vi "fetch_and_translate_trigger.vi"(8 "error in (no error)":errorcluster, 11 "AnalyserDL090624Scaffold in":refnum<class "AnalyserDL090624Scaffold.lvclass">) -> (0 "error out":errorcluster, 1 "sender TLC type":T1=enum."ImagingMode", 2 "trigger":T2, 3 "AnalyserDL090624Scaffold out":refnum<class "AnalyserDL090624Scaffold.lvclass">)   [LabVIEW 2010, in "AnalyserDL090624Scaffold.lvclass"]
uses:
  AnalyserDL090624Scaffold.lvclass
  internal_trigger_enum.ctl
  common/enumerations/top-level_component_type_enum.ctl
  common/classes/ErrorController/ErrorController/class_data.vi
  common/classes/ErrorController/ErrorController/ErrorController.lvclass
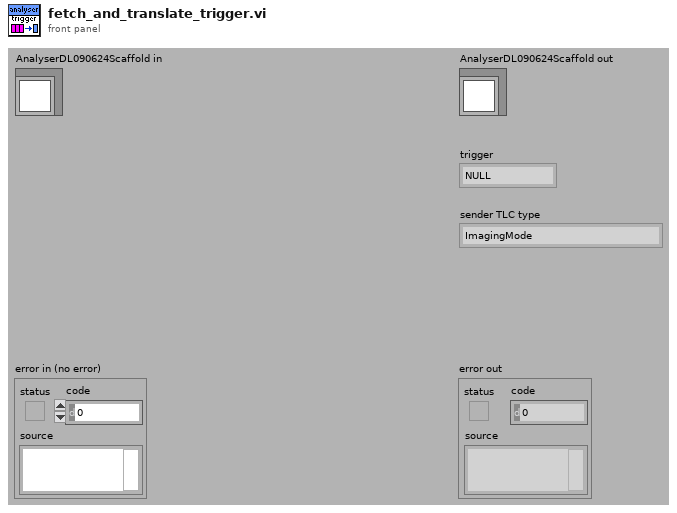
[diagram p1: front panel]
types:
  T1 = typedef "top-level_component_type_enum.ctl" = enum16{"undefined", "ImagingMode", "ScanHead", "DAQ", "ImageAssembler", "Display", "DataCollection", "Analyser", "Stimulator", "ExperimentController", "Instrument", "Stage"}
  T2 = typedef "AnalyserDL090624Scaffold.lvclass/internal_trigger_enum.ctl" = enum16{"NULL", "initialise", "terminate", "start", "stop", "analyse", "register as observer"}
  T3 = typedef "GenericToplevelComponent.lvclass/common_trigger_enum.ctl" = enum16{"NULL", "initialise", "terminate", "fetch command", "fetch data", "attach observer", "register as observer", "detach observer", "acknowledge", "start", "stop", "sweep started", "sweep finished", "experiment started", "experiment stopped"}
  T4 = typedef "trigger_type_enum.ctl" = enum8{"external", "internal", "common"}
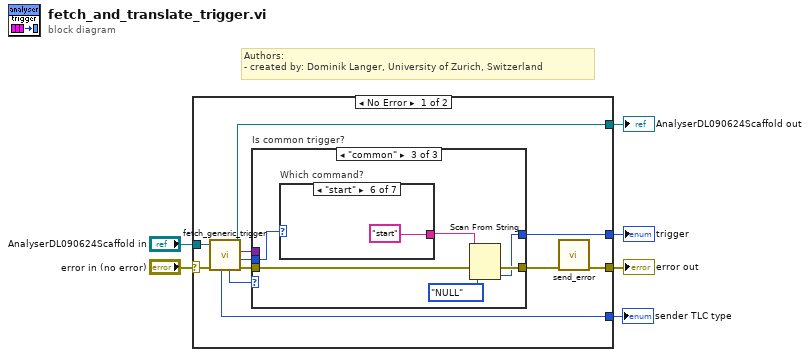
[diagram p0: block diagram]
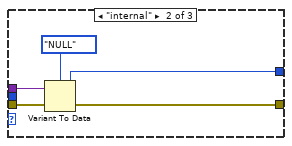
[diagram p3: hidden frame]
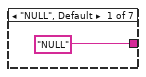
[diagram p4: hidden frame]
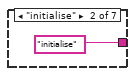
[diagram p5: hidden frame]
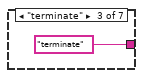
[diagram p6: hidden frame]
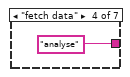
[diagram p7: hidden frame]
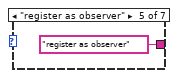
[diagram p8: hidden frame]
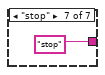
[diagram p9: hidden frame]
diagram:
  # "Authors: \n- created by: Dominik Langer, University of Zurich, Switzerland"
  n1 = case shown="No Error" "error in (no error)" {
    selector: "error in (no error)" -> [w16 w38]
    tunnel: [w9 w38] -> w5
    tunnel: [w14 w37] -> w3
    tunnel: "AnalyserDL090624Scaffold in" -> [w15 w37]
    tunnel: [w17 _] -> w1
    tunnel: [w7 _] -> w2
    frame No Error {
      n2 = call-dynamic "fetch_generic_trigger.vi"("error in (no error)"=w16, "GenericToplevelComponent in"=w15) -> ("error out"=w12:errorcluster, "common trigger"=w10:T3, "trigger"=w13:variant, "GenericToplevelComponent out"=w14:refnum<class "AnalyserDL090624Scaffold.lvclass">, "trigger type"=w11:T4, "sender TLC type"=w7:T1)  [unwired: 3 in, 1 out]
      n3 = case "Is common trigger?" shown="\"common\"" w11 {
        tunnel: w12 -> [w18 w23 w28]
        tunnel: w13 -> [_ w21 _]
        tunnel: w10 -> [_ _ w29]
        tunnel: [w18 w22 w27] -> w8
        tunnel: [_ w20 w24] -> w17
        frame "external", Default {
          # "No send_trigger.vi for GenericAnalyser!"
        }
        frame "internal" {
          n4 = Variant To Data(error in=w23, Variant=w21, type=internal_trigger_enum."NULL" ("trigger")) -> (error out=w22:errorcluster, data=w20:T2)
        }
        frame "common" {
          n5 = case "Which command?" shown="\"start\"" w29 {
            tunnel: ["NULL" "initialise" "terminate" "analyse" "register as observer" "start" "stop"] -> w26
            frame "NULL", Default {
            }
            frame "initialise" {
            }
            frame "terminate" {
            }
            frame "fetch data" {
            }
            frame "register as observer" {
            }
            frame "start" {
            }
            frame "stop" {
            }
          }
          n6 = Scan From String(input string=w26, error in=w28, default 1=internal_trigger_enum."NULL" ("trigger")) -> (error out=w27:errorcluster, output 1=w24:T2)  [unwired: 2 in, 2 out]
        }
      }
      n7 = call "send_error.vi"("error in (no error)"=w8) -> ("error out"=w9:errorcluster)  [unwired: 10 in]
    }
    frame Error {
    }
  }
  "error out" <- w5
  "AnalyserDL090624Scaffold out" <- w3
  "trigger" <- w1
  "sender TLC type" <- w2
